vi "Idle_GPIB2EthernetCommunicator.vi"(0 "String2Send":string=":slot 5;:temp:set 2.215000E+1", 1 "VISA resource name":refnum<visa-resource-name>="TCPIP0::192.168.0.100::1234::SOCKET", 3 "Delay Time (ms)":dbl=250.0 caption="Delay Time (s)", 4 "Bytes2Read":i32, 5 "ErrorIn":errorcluster) -> (14 "ReadBuffer":string, 19 "ErrorOut":errorcluster)   [LabVIEW 2012]
uses:
  <vilib>/Utility/error.llb/DialogType.ctl
panel:
  # ":slot 2;:ild:act?"
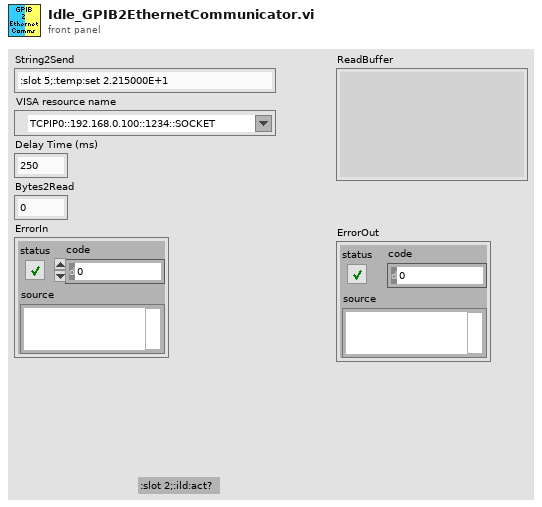
[diagram p1: front panel]
types:
  T1 = typedef "DialogType.ctl" = u16
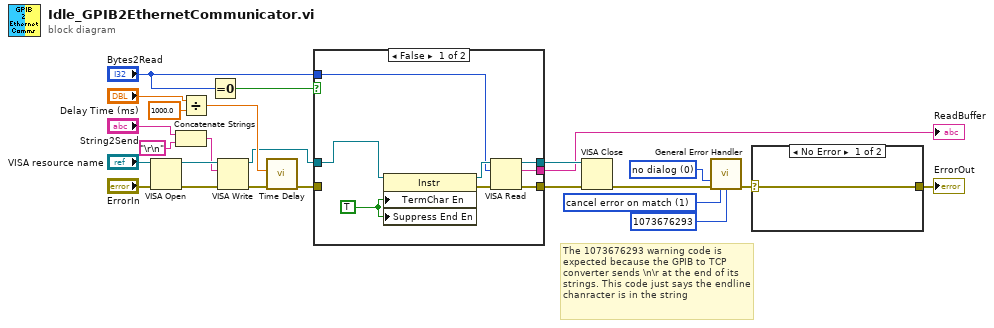
[diagram p0: block diagram]
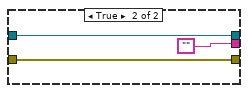
[diagram p2: hidden frame]
diagram:
  w10 = T1 0 items=["no dialog", "OK message", "continue or stop message", "OK message + warnings", "continue/stop + warnings"] ("type of dialog (OK msg:1)")
  w11 = 1 items=["no exception", "cancel error on match", "set error on match"] ("[exception action] (none:0)")
  # "The 1073676293 warning code is expected because the GPIB to TCP converter sends \\n\\r at the end of its strings. This code just says the endline chanracter is in the string"
  n1 = VISA Open(error in (no error)="ErrorIn", VISA resource name="VISA resource name") -> (VISA resource name=w21:refnum<visa-resource-name>, error out=w22:errorcluster)  [unwired: 3 in]
  n2 = Concatenate Strings("String2Send", "\r\n") -> (w18:string)
  n3 = Divide(x="Delay Time (ms)", y=1000.0) -> (x/y=w4:dbl)
  n4 = Equal To 0?(x="Bytes2Read") -> (x = 0?=w5:bool)
  n5 = VISA Write(VISA resource name=w21, write buffer=w18, error in (no error)=w22) -> (VISA resource name out=w1:refnum<visa-resource-name>, error out=w3:errorcluster)  [unwired: 1 out]
  n6 = call "Time Delay"("error in (no error)"=w3, "Delay Time (s)"=w4) -> ("error out"=w2:errorcluster)  [unwired: 9 in]
  n7 = case shown="False" w5 {
    tunnel: w2 -> [_ w34]
    tunnel: w1 -> [w25 w35]
    tunnel: [w29 w35] -> w15
    tunnel: [w28 w34] -> w14
    tunnel: [w27 ""] -> w13
    tunnel: "Bytes2Read" -> [w26 _]
    frame False {
      w32 = TRUE ("Message Based Settings:Termination Character Enable")
      n8 = property class="Instr"(reference=w25, "TermChar En"=w32, "Suppress End En"=w32) -> (reference out=w30:refnum<visa-resource-name>, error out=w31:errorcluster)  [unwired: 1 in]
      n9 = VISA Read(VISA resource name=w30, byte count=w26, error in (no error)=w31) -> (VISA resource name out=w29:refnum<visa-resource-name>, read buffer=w27:string, error out=w28:errorcluster)  [unwired: 1 out]
    }
    frame True {
    }
  }
  "ReadBuffer" <- w13
  n10 = VISA Close(VISA resource name=w15, error in (no error)=w14) -> (error out=w8:errorcluster)
  n11 = call <vilib>:"General Error Handler.vi"("type of dialog (OK msg:1)"=w10, "error in (no error)"=w8, "[exception action] (none:0)"=w11, "[exception code]"=1073676293) -> ("error out"=w7:errorcluster)  [unwired: 1 in, 10 out]
  n12 = case shown="No Error" w7 {
    selector: w7 -> [w36 w37]
    tunnel: [w36 w37] -> w12
    frame No Error {
    }
    frame Error {
    }
  }
  "ErrorOut" <- w12
